vi "rad_View Comparison Results.vi"(8 "error in (no error)":errorcluster, 9 "Files Found Only In New Image":path[](array[path]), 10 "Files Found Only In Original Image":path[](array[path]), 11 "Modified Files":path[](array[path])) -> (0 "error out":errorcluster)   [LabVIEW 2016]
uses:
  <vilib>/Utility/miscctls.llb/LVRowAndColumnTypeDef.ctl
panel:
  in  "Log Results":bool
  in  "OK":bool
  in  "Results Table":i32(listbox)
  # "Image differences are listed below..."
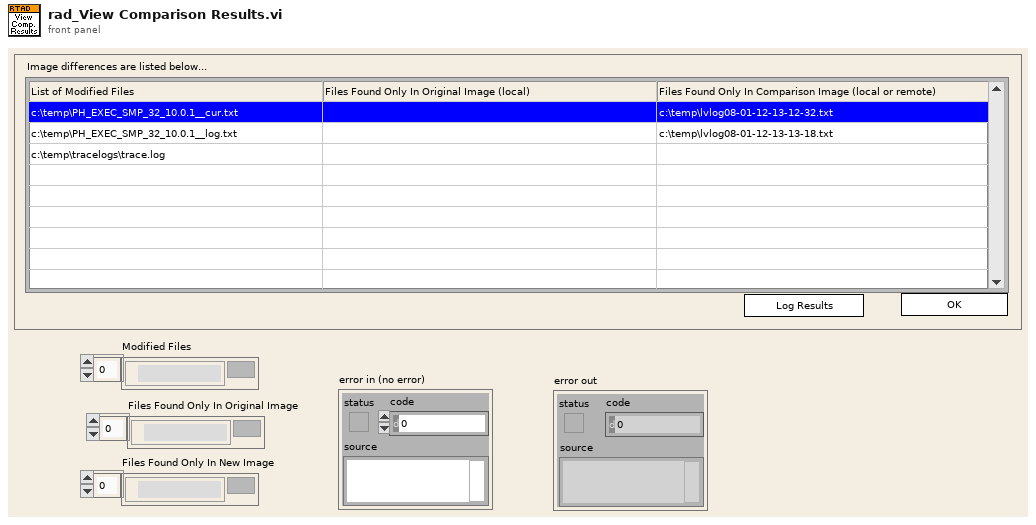
[diagram p1: front panel]
types:
  T1 = typedef "LVRowAndColumnTypeDef.ctl" = cluster{"Row":i32, "Column":i32}
  T2 = enum16{"open", "replace", "create", "open or create", "replace or create", "replace or create with confirmation"}
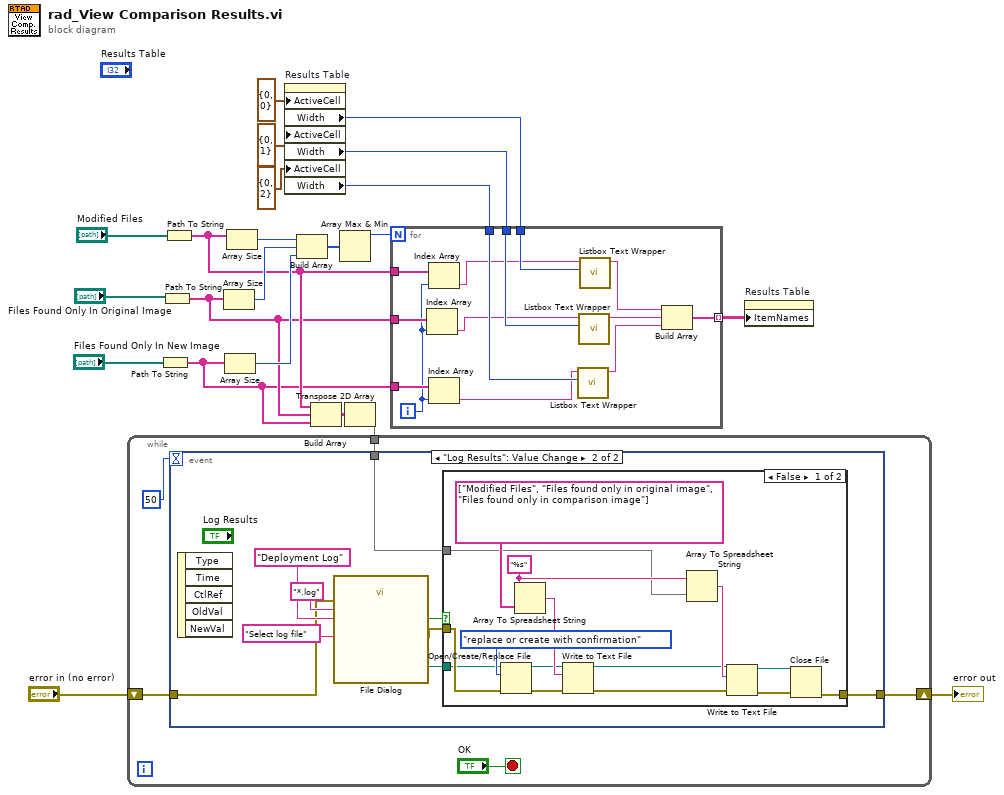
[diagram p0: block diagram]
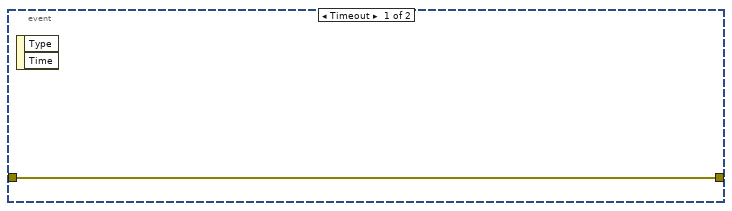
[diagram p2: hidden frame]
diagram:
  n1 = Path To String(path="Files Found Only In New Image") -> (string=w3:string[])
  n2 = Path To String(path="Files Found Only In Original Image") -> (string=w4:string[])
  n3 = Path To String(path="Modified Files") -> (string=w5:string[])
  n4 = Array Size(array=w4) -> (size(s)=w21:i32)
  n5 = Array Size(array=w3) -> (size(s)=w20:i32)
  n6 = Array Size(array=w5) -> (size(s)=w22:i32)
  n7 = property on="Results Table" class="MCListbox (strict)"("ActiveCell"=T1 {"Row"=0, "Column"=0} ("Active Cell:Active Cell"), "ActiveCell"=T1 {"Row"=0, "Column"=1} ("Active Cell:Active Cell"), "ActiveCell"=T1 {"Row"=0, "Column"=2} ("Active Cell:Active Cell")) -> ("Width"=w11:u32, "Width"=w10:u32, "Width"=w9:u32)  [unwired: 2 in, 2 out]
  n8 = Build Array(w22, w21, w20) -> (w19:i32[])
  n9 = Build Array(w5, w4, w3) -> (w2:string[][])
  n10 = Array Max & Min(array=w19) -> (max value=w18:i32)  [unwired: 3 out]
  n11 = Transpose 2D Array(2D array=w2) -> (transposed array=w1:string[][])
  n12 = while {
    shift-right: [w25] -> w6
    shift-left: "error in (no error)" -> [w24]
    tunnel: w1 -> [w23]
    stop <- "OK" stop-if-true
    n13 = event shown="[1] \"Log Results\": Value Change" {
      selector: _ -> [_ _]
      dyn-events: _ -> [_ _]
      timeout: 50 -> [_ _]
      tunnel: [w28 w34] -> w25
      tunnel: w24 -> [w28 w33]
      tunnel: w23 -> [_ w29]
      event Timeout {
        n14 = event-data() -> ()  [unwired: 1 in, 2 out]
      }
      event "Log Results": Value Change {
        n15 = event-data() -> ()  [unwired: 1 in, 5 out]
        n16 = call "File Dialog"("prompt"="Select log file", "error in"=w33, "pattern (all files)"="*.log", "pattern label"="Deployment Log") -> ("selected path"=w30:path, "cancelled"=w31:bool, "error out"=w32:errorcluster)  [unwired: 3 in, 6 out]
        n17 = case shown="False" w31 {
          tunnel: [w41 w53] -> w34
          tunnel: w32 -> [w40 w53]
          tunnel: w30 -> [w39 _]
          tunnel: w29 -> [w38 _]
          frame False {
            w47 = "%s" ("format string")
            n18 = Open/Create/Replace File(file path (use dialog)=w39, error in=w40, operation (0:open)=T2."replace or create with confirmation") -> (refnum out=w49:refnum<file>, error out=w48:errorcluster)  [unwired: 4 out]
            n19 = Array To Spreadsheet String(array=string[] ["Modified Files", "Files found only in original image", "Files found only in comparison image"], 3:w47) -> (spreadsheet string=w50:string)  [unwired: 1 out]
            n20 = Write to Text File(file (use dialog)=w49, text=w50, error in=w48) -> (refnum out=w45:refnum<file>, error out=w44:errorcluster)  [unwired: 2 out]
            n21 = Array To Spreadsheet String(array=w38, 3:w47) -> (spreadsheet string=w46:string)  [unwired: 1 out]
            n22 = Write to Text File(file (use dialog)=w45, text=w46, error in=w44) -> (refnum out=w42:refnum<file>, error out=w43:errorcluster)  [unwired: 2 out]
            n23 = Close File(refnum=w42, error in=w43) -> (error out=w41:errorcluster)  [unwired: 1 out]
          }
          frame True {
          }
        }
      }
    }
  }
  "error out" <- w6
  n24 = for {
    N: w18 -> [_]
    tunnel: w5 -> [w67]
    tunnel: w4 -> [w66]
    tunnel: w3 -> [w65]
    tunnel: [w63] -> w8 mode=indexing
    tunnel: w11 -> [w62]
    tunnel: w10 -> [w61]
    tunnel: w9 -> [w60]
    i -> [w64]
    n25 = Index Array(array=w66, index=w64) -> (element=w58:string)
    n26 = Index Array(array=w67, index=w64) -> (element=w59:string)
    n27 = Index Array(array=w65, index=w64) -> (element=w57:string)
    n28 = call "Listbox Text Wrapper.vi"("Size:Width"=w60, "Input Text"=w57) -> ("Wrapped Text"=w56:string)  [unwired: 9 in]
    n29 = call "Listbox Text Wrapper.vi"("Size:Width"=w61, "Input Text"=w58) -> ("Wrapped Text"=w55:string)  [unwired: 9 in]
    n30 = call "Listbox Text Wrapper.vi"("Size:Width"=w62, "Input Text"=w59) -> ("Wrapped Text"=w54:string)  [unwired: 9 in]
    n31 = Build Array(w54, w55, w56) -> (w63:string[])
  }
  n32 = property on="Results Table" class="MCListbox (strict)"("ItemNames"=w8) -> ()  [unwired: 2 in, 2 out]
